vi "BinAvgRef.vi"(6 "X ref array":dbl[](array[numeric]), 7 "Extend to 0":bool, 9 "X coumn index":i32, 10 "Bin size":dbl, 11 "Data in":dbl[][](array[numeric])) -> (2 "Binned data down":dbl[][](array[numeric]), 3 "Binned data up":dbl[][](array[numeric]))   [LabVIEW 2016]
panel:
  out "Waveform Graph 3":dbl[][](graph)
  out "Waveform Graph 2":dbl[][](graph)
  out "Waveform Graph":dbl[][](graph)
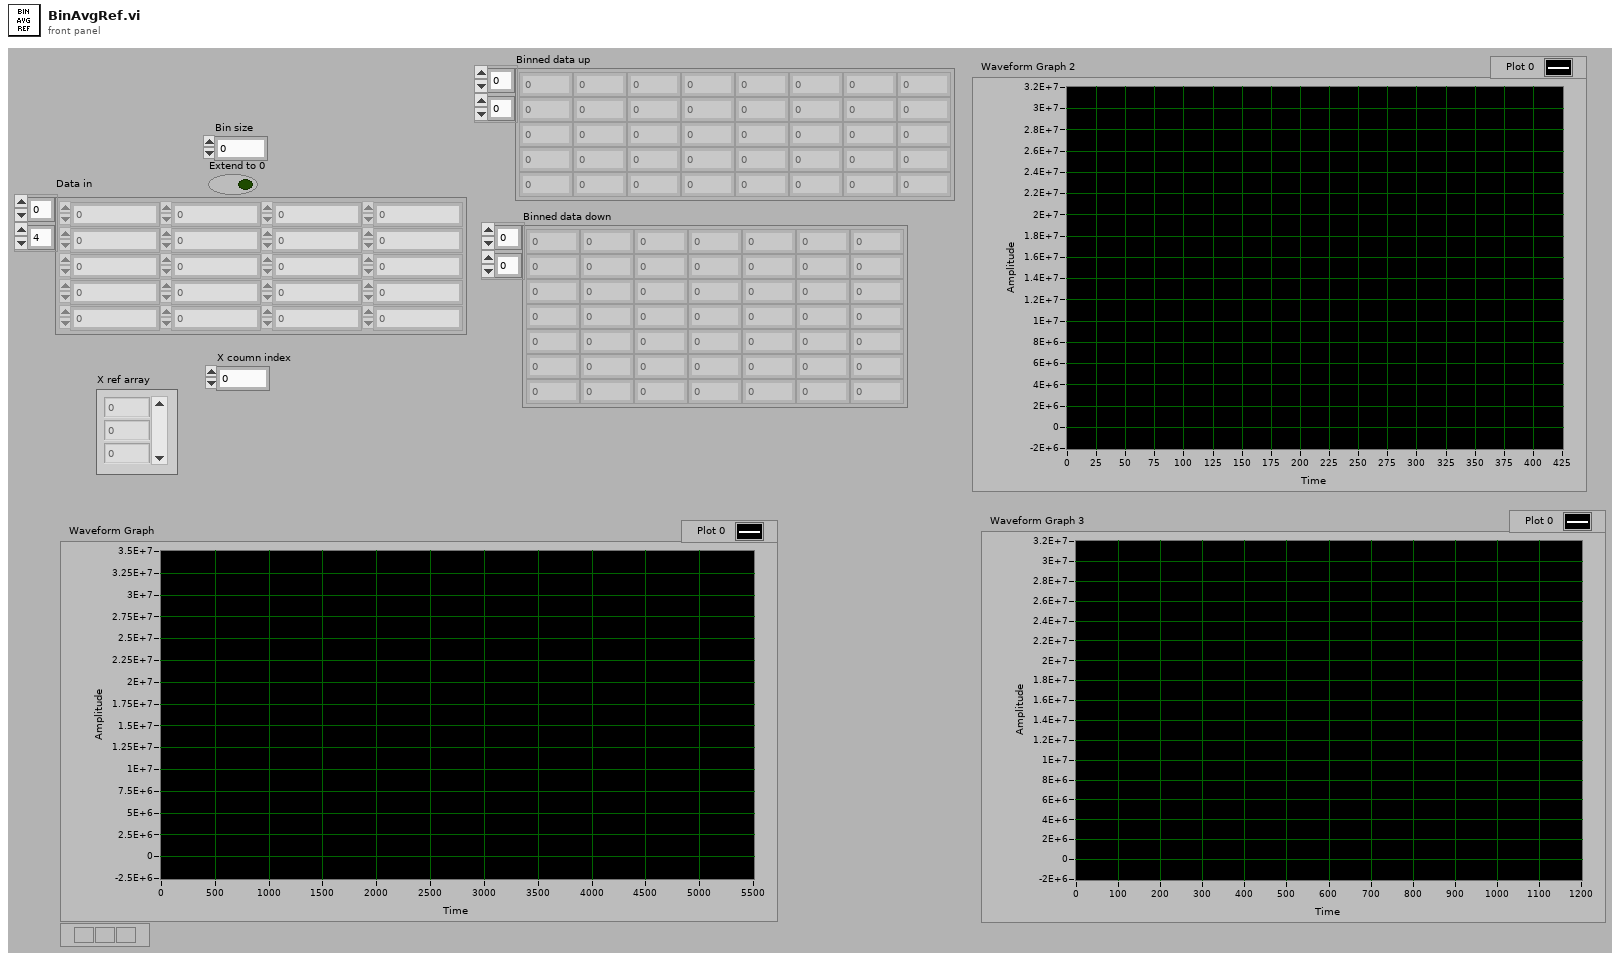
[diagram p1: front panel]
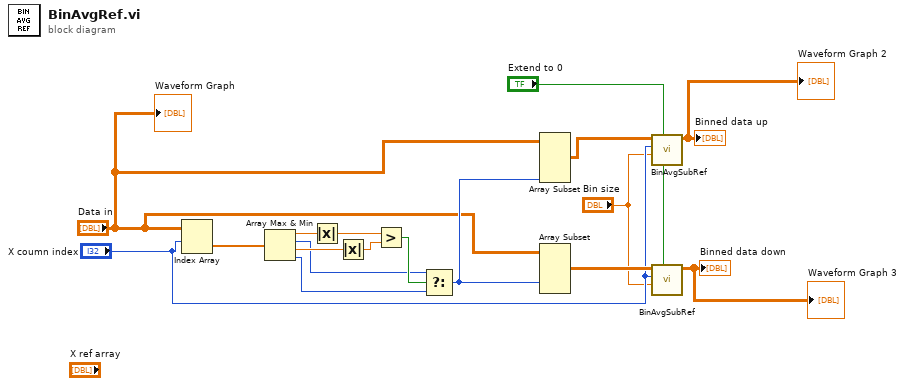
[diagram p0: block diagram]
diagram:
  n1 = Index Array(array="Data in", index (row)="X coumn index") -> (element=w17:dbl[])  [unwired: 1 in]
  n2 = Array Max & Min(array=w17) -> (max value=w16:dbl, max index (indices)=w11:i32, min value=w15:dbl, min index (indices)=w10:i32)
  n3 = Absolute Value(x=w16) -> (abs(x)=w13:dbl)
  n4 = Absolute Value(x=w15) -> (abs(x)=w14:dbl)
  n5 = Greater?(x=w13, y=w14) -> (0:w12:bool)
  n6 = Select(t=w11, s=w12, f=w10) -> (s? t:f=w4:i32)
  n7 = Array Subset(array="Data in", length (col)=w4) -> (w9:dbl[][])  [unwired: 3 in]
  n8 = Array Subset(array="Data in", index (col)=w4) -> (w8:dbl[][])  [unwired: 3 in]
  n9 = call "BinAvgSubRef.vi"("Extend to 0"="Extend to 0", "Bin size"="Bin size", "X coumn index"="X coumn index", "Data in"=w9) -> ("Binned data"=→"Binned data up" →"Waveform Graph 2":dbl[][])  [unwired: 7 in]
  n10 = call "BinAvgSubRef.vi"("Extend to 0"="Extend to 0", "Bin size"="Bin size", "X coumn index"="X coumn index", "Data in"=w8) -> ("Binned data"=→"Binned data down" →"Waveform Graph 3":dbl[][])  [unwired: 7 in]
  "Waveform Graph" <- "Data in"
